vi "temp_ctr.vi"() -> ()   [LabVIEW 2011]
uses:
  multi_queue_enum.ctl
  <vilib>/Instr/_visa.llb/VISA Configure Serial Port (Instr).vi
panel:
  out "time 2":timestamp
  out "data":dbl[](array[numeric])
  out "time":timestamp
  in  "deg":dbl
  in  "ch":u8
  in  "stop":bool
  in  "write":bool
  in  "val":T1={"error in (no error)"={"status"=FALSE, "code"=0, "source"=""}, "ser"={"baud rate (9600)"=9600, "timeout (10sec)"=10000, "data bits (8)"=8, "stop bits (10: 1 bit)"=10, "parity (0:none)"=enum."None", "VISA resource name"=""}, "init?"=FALSE} {"ser"."stop bits (10: 1 bit)" items=["1.0"=10, "1.5"=15, "2.0"=20]; "ser"."data bits (8)" min=5 max=8 step=1}
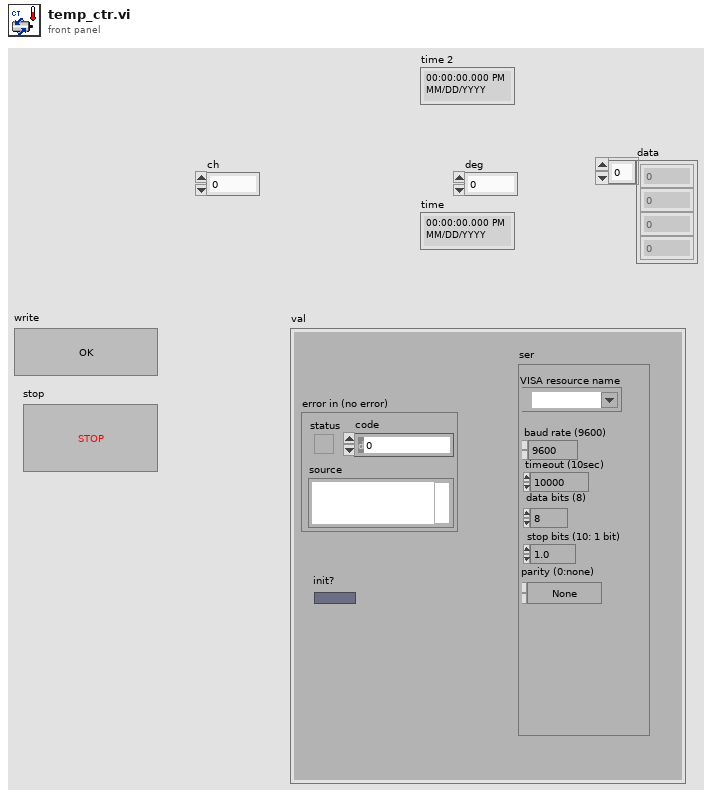
[diagram p1: front panel]
types:
  T1 = cluster{"error in (no error)":errorcluster, "ser":cluster{"baud rate (9600)":u32, "timeout (10sec)":u32, "data bits (8)":u16, "stop bits (10: 1 bit)":u16, "parity (0:none)":enum16{"None", "Odd", "Even", "Mark", "Space"}, "VISA resource name":refnum<visa-resource-name>}, "init?":bool}
  T2 = typedef "multi_queue_enum.ctl" = enum16{"Noop", "add queues", "Send Pro1", "Send data", "Get Pro1", "Get data", "Flush Pro1", "Flush data", "Destroy Pro1", "Destroy data"}
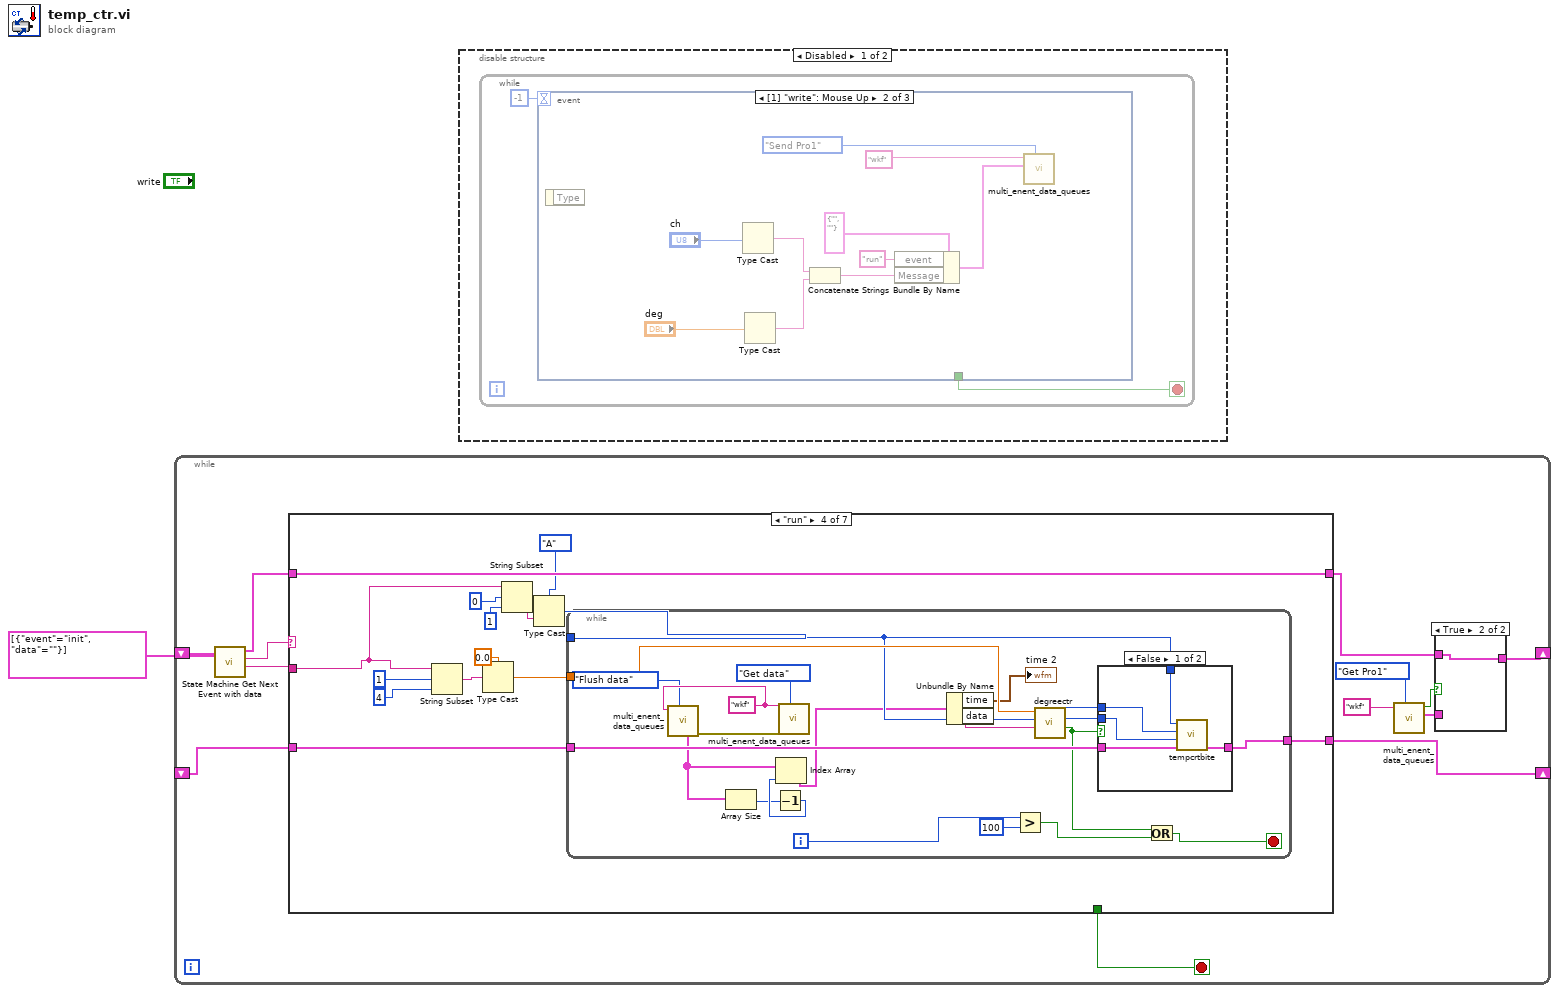
[diagram p0: block diagram]
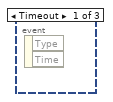
[diagram p2: hidden frame]
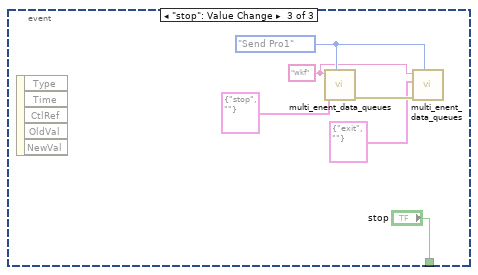
[diagram p3: hidden frame]
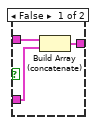
[diagram p5: hidden frame]
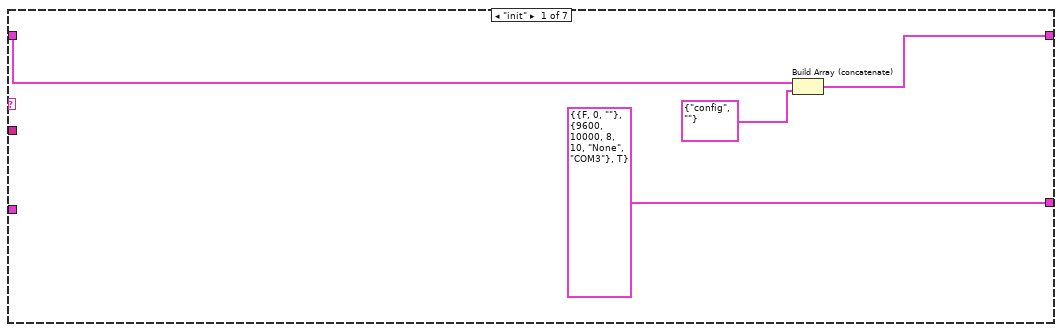
[diagram p6: hidden frame]
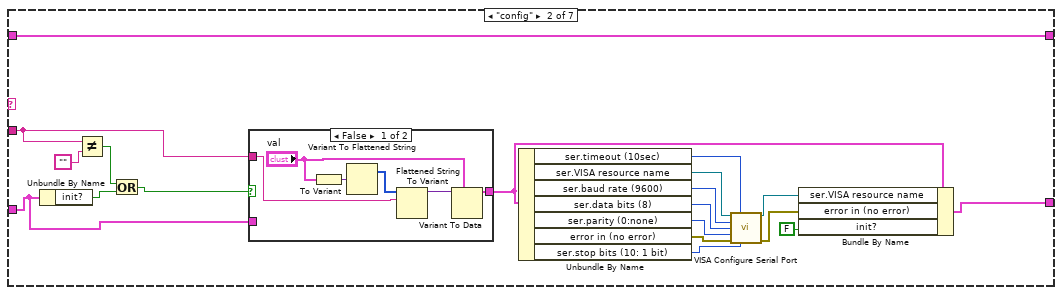
[diagram p7: hidden frame]
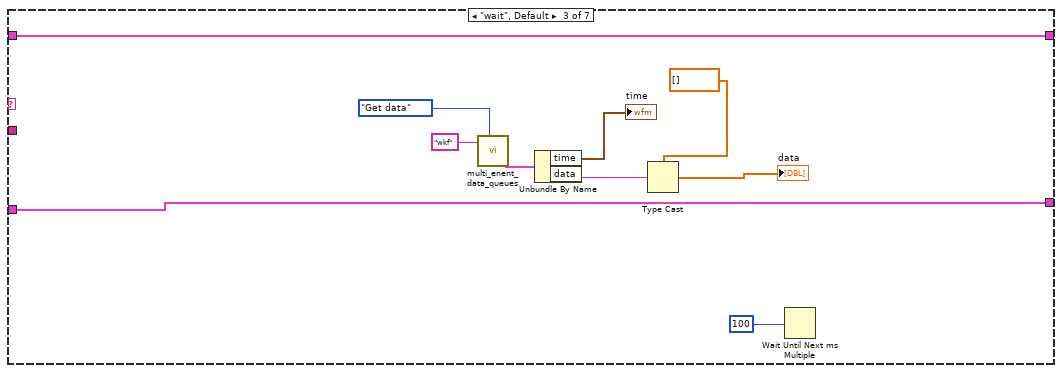
[diagram p9: hidden frame]
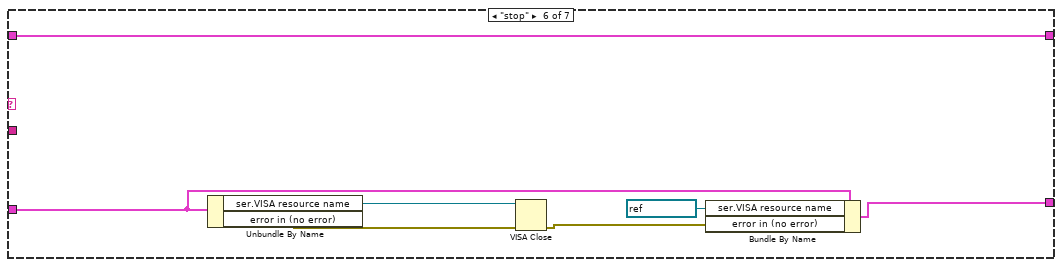
[diagram p12: hidden frame]
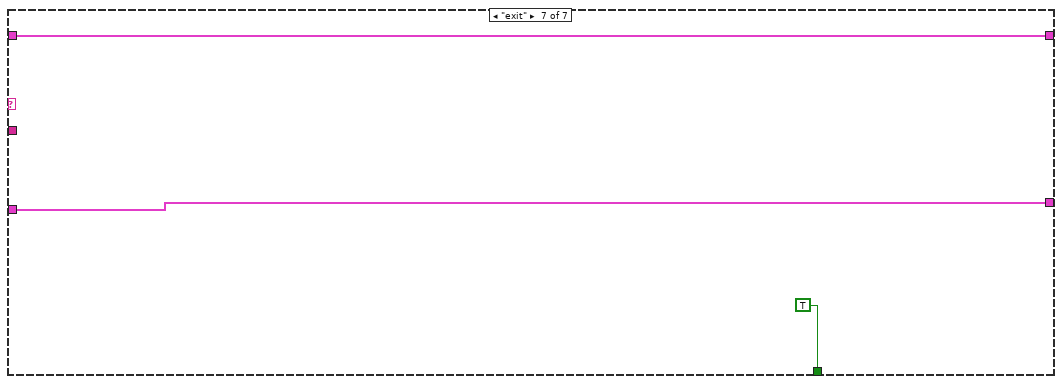
[diagram p13: hidden frame]
diagram:
  n1 = while {
    shift-right: [w4] -> _
    shift-left: cluster{"event":string, "data":string}[] [{"event"="init", "data"=""}] ("enent data queue in") -> [w14]
    shift-right: [w9] -> _
    shift-left: _ -> [w8]
    stop <- w10 stop-if-true
    n2 = call "State Machine Get Next Event with data.vi"("enent data queue in"=w14) -> ("data"=w11:string, "next event"=w12:string, "event queue out"=w13:cluster{"event":string, "data":string}[])  [unwired: 4 in]
    n3 = case shown="\"run\"" w12 {
      tunnel: w13 -> [w22 w41 w58 w72 w101 w102 w109]
      tunnel: w11 -> [_ w30 _ w71 _ _ _]
      tunnel: [w21 w41 w58 w72 w101 w102 w109] -> w5
      tunnel: [_ _ _ _ _ _ TRUE] -> w10
      tunnel: [T1 {"error in (no error)"={"status"=FALSE, "code"=0, "source"=""}, "ser"={"baud rate (9600)"=9600, "timeout (10sec)"=10000, "data bits (8)"=8, "stop bits (10: 1 bit)"=10, "parity (0:none)"=enum."None", "VISA resource name"="COM3"}, "init?"=TRUE} ("val") w33 w57 w63 w100 w104 w110] -> w9
      tunnel: w8 -> [_ w27 w57 w62 w100 w107 w110]
      frame "init" {
        n4 = Build Array (concatenate)(w22, cluster{"event":string, "data":string} {"event"="config", "data"=""} ("enent data queue in")) -> (w21:cluster{"event":string, "data":string}[])
      }
      frame "config" {
        n5 = Unbundle By Name(w27) -> ("init?"=w25:bool)
        n6 = Not Equal?(x=w30, y="") -> (x != y?=w24:bool)
        n7 = Or(x=w24, y=w25) -> (x .or. y?=w23:bool)
        n8 = case shown="False" w23 {
          tunnel: [w47 w48] -> w26
          tunnel: w30 -> [w46 _]
          tunnel: w27 -> [_ w48]
          frame False {
            n9 = To Variant(anything="val") -> (Variant=w42:variant)
            n10 = Variant To Flattened String(Variant=w42) -> (1:w44:i16[])  [unwired: 1 out]
            n11 = Flattened String To Variant(6:w46, 7:w44) -> (3:w45:variant)  [unwired: 1 in, 1 out]
            n12 = Variant To Data(type="val", Variant=w45) -> (data=w47:T1)  [unwired: 1 in, 1 out]
          }
          frame True {
          }
        }
        n13 = Unbundle By Name(w26) -> ("ser.timeout (10sec)"=w34:u32, "ser.VISA resource name"=w40:refnum<visa-resource-name>, "ser.baud rate (9600)"=w39:u32, "ser.data bits (8)"=w38:u16, "ser.parity (0:none)"=w37:enum16{"None", "Odd", "Even", "Mark", "Space"}, "error in (no error)"=w36:errorcluster, "ser.stop bits (10: 1 bit)"=w35:u16)
        n14 = call-poly "VISA Configure Serial Port"("VISA resource name"=w40, "timeout (10sec)"=w34, "baud rate (9600)"=w39, "data bits (8)"=w38, "parity (0:none)"=w37, "error in (no error)"=w36, "stop bits (10: 1 bit)"=w35) -> ("VISA resource name out"=w32:refnum<visa-resource-name>, "error out"=w28:errorcluster)  [unwired: 7 in]
        n15 = Bundle By Name(cluster=w26, "ser.VISA resource name"=w32, "error in (no error)"=w28, "init?"=FALSE) -> (w33:T1)
      }
      frame "wait", Default {
        n16 = call "multi_enent_data_queues.vi"("Mode"=multi_queue_enum."Get data", "name"="wkf") -> ("data 2"=w53:cluster{"time":timestamp, "data":string})  [unwired: 5 in, 4 out]
        n17 = Unbundle By Name(w53) -> ("time"=→"time":timestamp, "data"=w51:string)
        n18 = Type Cast(type=dbl[] [], x=w51) -> (*(type *) &x=→"data":dbl[])
        n19 = Wait Until Next ms Multiple(millisecond multiple=u32 100) -> ()  [unwired: 1 out]
      }
      frame "run" {
        n20 = String Subset(string=w71, offset (0)=1, length (rest)=4 ("length (rest)")) -> (substring=w66:string)
        n21 = Type Cast(type=0.0 ("deg"), x=w66) -> (*(type *) &x=w59:dbl)
        n22 = String Subset(string=w71, offset (0)=0, length (rest)=1 ("length (rest)")) -> (substring=w64:string)
        n23 = Type Cast(type=enum8{"A", "B"}."A" ("ID"), x=w64) -> (*(type *) &x=w60:enum8{"A", "B"})
        n24 = while {
          tunnel: [w93] -> w63
          tunnel: w62 -> [w92]
          tunnel: w60 -> [w90]
          tunnel: w59 -> [w91]
          i -> [w86]
          stop <- w82 stop-if-true
          w79 = "wkf" ("name")
          n25 = call "multi_enent_data_queues.vi"("Mode"=multi_queue_enum."Flush data", "name"=w79) -> ("error out"=w77:errorcluster, "remaining elements"=w76:cluster{"time":timestamp, "data":string}[])  [unwired: 5 in, 3 out]
          n26 = Array Size(array=w76) -> (size(s)=w74:i32)
          n27 = Decrement(x=w74) -> (x-1=w75:i32)
          n28 = Index Array(array=w76, index=w75) -> (element=w73:cluster{"time":timestamp, "data":string})
          n29 = call "multi_enent_data_queues.vi"("Mode"=multi_queue_enum."Get data", "error in"=w77, "name"=w79) -> ()  [unwired: 4 in, 5 out]
          n30 = Unbundle By Name(w73) -> ("time"=→"time 2":timestamp, "data"=w89:string)
          n31 = Greater?(x=w86, y=100) -> (0:w84:bool)
          n32 = call "degreectr.vi"("testdata"=w89, "ID"=w90, "deg"=w91) -> ("stop"=w83:bool, "pulse"=w88:u16, "方向"=w87:enum8{"正转", "反转\n"})  [unwired: 6 in]
          n33 = case shown="False" w83 {
            tunnel: [w98 w99] -> w93
            tunnel: w92 -> [w97 w99]
            tunnel: w90 -> [w96 _]
            tunnel: w88 -> [w95 _]
            tunnel: w87 -> [w94 _]
            frame False {
              n34 = call "tempcrtbite.vi"("input"=w97, "pulse"=w95, "方向"=w94, "ID"=w96) -> ("output"=w98:T1)  [unwired: 7 in]
            }
            frame True {
            }
          }
          n35 = Or(x=w83, y=w84) -> (x .or. y?=w82:bool)
        }
      }
      frame "pid" {
      }
      frame "stop" {
        n36 = Unbundle By Name(w107) -> ("ser.VISA resource name"=w106:refnum<visa-resource-name>, "error in (no error)"=w108:errorcluster)
        n37 = VISA Close(VISA resource name=w106, error in (no error)=w108) -> (error out=w105:errorcluster)
        n38 = Bundle By Name(cluster=w107, "ser.VISA resource name"=refnum<visa-resource-name> refnum, "error in (no error)"=w105) -> (w104:T1)
      }
      frame "exit" {
      }
    }
    n39 = call "multi_enent_data_queues.vi"("Mode"=multi_queue_enum."Get Pro1", "name"="wkf") -> ("process"=w3:cluster{"event":string, "par":string}, "timed out?"=w2:bool)  [unwired: 5 in, 3 out]
    n40 = case shown="True" w2 {
      tunnel: w5 -> [w17 w18]
      tunnel: [w16 w18] -> w4
      tunnel: w3 -> [w15 _]
      frame False {
        n41 = Build Array (concatenate)(w17, w15) -> (w16:cluster{"event":string, "par":string}[])
      }
      frame True {
      }
    }
  }
  n42 = disable-structure shown="Disabled" {
    frame Disabled {
      n43 = while {
        stop <- w112 stop-if-true
        n44 = event shown="[1] \"write\": Mouse Up" {
          selector: _ -> [_ _ _]
          dyn-events: _ -> [_ _ _]
          timeout: -1 -> [_ _ _]
          tunnel: [_ _ "stop"] -> w112
          event Timeout {
            n45 = event-data() -> ()  [unwired: 1 in, 2 out]
          }
          event "write": Mouse Up {
            n46 = event-data() -> ()  [unwired: 1 in, 1 out]
            n47 = Type Cast(x="ch") -> (*(type *) &x=w116:string)  [unwired: 1 in]
            n48 = Type Cast(x="deg") -> (*(type *) &x=w114:string)  [unwired: 1 in]
            n49 = Concatenate Strings(w116, w114) -> (w115:string)
            n50 = Bundle By Name(cluster=cluster{"event":string, "Message":string} {"event"="", "Message"=""} ("process"), "event"="run", "Message"=w115) -> (w120:cluster{"event":string, "Message":string})
            n51 = call "multi_enent_data_queues.vi"("Mode"=multi_queue_enum."Send Pro1", "process"=w120, "name"="wkf") -> ()  [unwired: 4 in, 5 out]
          }
          event "stop": Value Change {
            w125 = "wkf" ("name")
            w126 = multi_queue_enum."Send Pro1" ("Mode")
            n52 = event-data() -> ()  [unwired: 1 in, 5 out]
            n53 = call "multi_enent_data_queues.vi"("Mode"=w126, "process"=cluster{"event":string, "Message":string} {"event"="stop", "Message"=""}, "name"=w125) -> ("error out"=w127:errorcluster)  [unwired: 4 in, 4 out]
            n54 = call "multi_enent_data_queues.vi"("Mode"=w126, "error in"=w127, "process"=cluster{"event":string, "Message":string} {"event"="exit", "Message"=""}, "name"=w125) -> ()  [unwired: 3 in, 5 out]
          }
        }
      }
    }
    frame Enabled {
    }
  }
